vi "SigGen-Compute Max Level (wrapper).vi"(0 "Stimulus Channel":T22(xcontrol), 7 "Sampling Rate (Hz)":dbl, 9 "Npts":i32, 11 "error in (no error)":errorcluster) -> (4 "Stimulus Channel out":T22(xcontrol), 14 "Max Level":dbl, 15 "error out":errorcluster)   [LabVIEW 2020]
uses:
  Controls/Stimulus Channel XCtl/Stimulus Channel.xctl
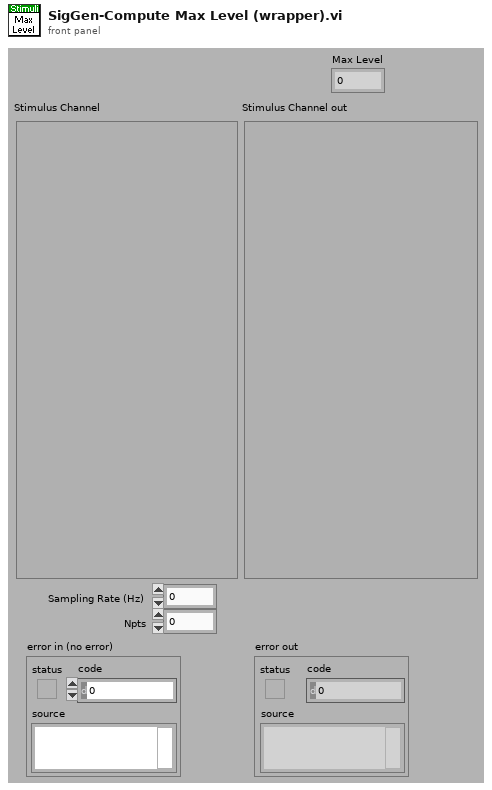
[diagram p1: front panel]
types:
  T1 = typedef "Waveform XCtl.xctl/Waveform Data.ctl" = cluster{"Type":T2, "Tone":T3, "Pulse Train":T4, "Noise":T7, "File":T8, "FMSweep":T9, "Chirp Train":T10, "Complex Tone":cluster{"Params":T12, "Data":T14}, "Moving Ripple":T15}
  T2 = typedef "Waveform Enum.ctl" = enum16{"OFF", "Tone", "Noise", "Pulse Train", "File", "FM Sweep", "Chirp Train", "Complex Tone", "FM Tone", "Moving Ripple"}
  T3 = typedef "Tone Params.ctl" = cluster{"Frequency (kHz)":dbl, "Last Freq":dbl, "Last Phase":dbl}
  T4 = typedef "Pulse Train Params.ctl" = cluster{"Pulse width (us)":dbl, "Pulse rate (Hz)":dbl, "Gap (ms)":dbl, "Polarity":T5, "PT State":T6, "Asynch":bool}
  T5 = typedef "Pulse Polarity.ctl" = enum16{"POS", "NEG", "POS-NEG", "NEG-POS"}
  T6 = typedef "PT-Continuous State.ctl" = cluster{"Template":dbl[], "Nperiod":i32, "Index":i32, "Pulse Rate (Hz)":dbl, "Phase (cycles)":dbl, "Noff":i32}
  T7 = typedef "Noise Params.ctl" = cluster{"InvFilt":bool, "Noise":dbl[], "CurPt":i32, "Aweight":bool, "Seed":i32, "afile":path}
  T8 = typedef "StimFile-Params.ctl" = cluster{"Filename":path, "Signal":dbl[], "Channel":i32, "stream":bool, "offset":i32, "nreps":i32, "loops":i32, "Randomize":bool, "order":i32[], "Seed":i32, "Tokens":i32}
  T9 = typedef "FM Sweep Params.ctl" = cluster{"Rate (oct/s)":dbl, "Fmin (Hz)":dbl, "Fmax (Hz)":dbl, "Ramp (ms)":dbl, "Linear":bool}
  T10 = typedef "Chirp Train.ctl" = cluster{"Params":T11, "Data":cluster{"WF":dbl[]}}
  T11 = typedef "Chirp Train Params.ctl" = cluster{"Fmin (kHz)":dbl, "Fmax (kHz)":dbl, "Compensate":bool, "Duration (ms)":dbl}
  T12 = typedef "CT-Params.ctl" = cluster{"F0 (Hz)":dbl, "Band":cluster{"Flow (Hz)":dbl, "Fhigh (Hz)":dbl}, "Phase":T13, "Min F0 (Hz)":dbl, "Max F0 (Hz)":dbl, "ContinRandPhase":bool, "Max peak factor":dbl, "Max mod depth":dbl, "MinHarmNum":i32, "MaxHarmNum":i32, "Level Mode":enum16{"per component", "overall rms"}, "% jitter":dbl}
  T13 = typedef "CT-Phase Enum.ctl" = enum16{"Cosine", "Random", "Alternating"}
  T14 = typedef "CT-Runtime Data.ctl" = cluster{"Ncomp":i32, "MinHarm":i32, "Phase":dbl[], "Amplitude":dbl[], "Npts/frame":i32, "Last F0":dbl, "Fmin":dbl, "Fmax":dbl, "Lslope":dbl, "randphase":bool, "overall rms":bool, "fmult":dbl[], "jittered":bool}
  T15 = typedef "Moving Ripple.ctl" = cluster{"Params":T16, "Data":T17}
  T16 = typedef "Moving Ripple.Params.ctl" = cluster{"Fmin":dbl, "Fmax":dbl, "Density":dbl, "Velocity":dbl, "Depth":dbl, "Phase":dbl, "Comp/oct":i32}
  T17 = typedef "Moving Ripple.Data.ctl" = cluster{"Freq":dbl[], "A":dbl[], "phase":dbl[], "Phase":dbl}
  T18 = typedef "Filter XCtl.xctl/Filter Data.ctl" = cluster{"CF (kHz)":dbl, "BW (kHz)":dbl, "IIR Filter Cluster":cluster{"filter structure":enum32{"IIR 2nd Order", "IIR 4th Order"}, "Reverse Coefficients":dbl[], "Forward Coefficients":dbl[]}, "Final Filter State":dbl[], "Scale Factor":dbl, "Final Filter State 2":dbl[], "Quadrature":bool, "Type":enum16{"Lowpass", "Highpass", "Bandpass", "Bandstop", "OFF"}}
  T19 = typedef "Gate Control.xctl/Gate Data.ctl" = cluster{"Active":bool, "Delay (ms)":dbl, "Width (ms)":dbl, "Ramp (ms)":dbl}
  T20 = typedef "Level XCtl.xctl/Level Data.ctl" = cluster{"Level":dbl, "Units":T21, "Max":dbl, "Multiplier":dbl, "Cal File":path, "Cal":cluster{"Freq (Hz)":dbl[], "Mag (dB SPL)":dbl[], "Phase (deg)":dbl[]}}
  T21 = typedef "Level Units.ctl" = enum16{"dB atten", "dB SPL", "dB re 1 Vrms", "dB V/Hz½", "mW", "dB HL", "Volts", "dB mW"}
  T22 = cluster{"Waveform":T1, "Filter":T18, "Gate":T19, "Level":T20}
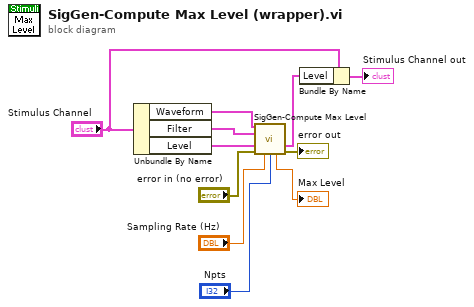
[diagram p0: block diagram]
diagram:
  n1 = Unbundle By Name("Stimulus Channel") -> ("Waveform"=w2:T1, "Filter"=w1:T18, "Level"=w11:T20)
  n2 = call "SigGen-Compute Max Level.vi"("Waveform"=w2, "Filter XCtl"=w1, "Level"=w11, "error in (no error)"="error in (no error)", "Sampling Rate (Hz)"="Sampling Rate (Hz)", "Npts"="Npts") -> ("Level out"=w5:T20, "Max Level"=→"Max Level":dbl, "error out"=→"error out":errorcluster)  [unwired: 7 in]
  n3 = Bundle By Name(cluster="Stimulus Channel", "Level"=w5) -> (→"Stimulus Channel out":T22)
